vi "CloseAllGrips.vi"(8 "error in (no error)":errorcluster) -> (0 "error out":errorcluster)   [LabVIEW 2017]
uses:
  Projekt-RubikLibrary/RubikLibraryRT.lvlib
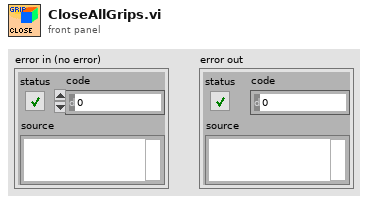
[diagram p1: front panel]
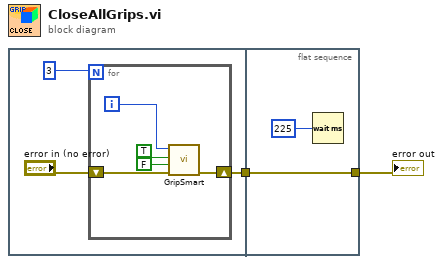
[diagram p0: block diagram]
diagram:
  n1 = flat-sequence {
    tunnel: [w5] -> w1
    tunnel: [w12] -> w2
    tunnel: w1 -> [w12]
    frame #0 {
      n2 = for {
        N: 3 -> [_]
        shift-right: [w9] -> w5
        shift-left: "error in (no error)" -> [w10]
        i -> [w6]
        n3 = call "GripSmart.vi"("error in"=w10, "NoWait"=FALSE, "Grip closed (in)"=TRUE, "Servo"=w6) -> ("error out"=w9:errorcluster)  [unwired: 6 in, 1 out]
      }
    }
    frame #1 {
      n4 = Wait (ms)(milliseconds to wait=u32 225) -> ()  [unwired: 1 out]
    }
  }
  "error out" <- w2
